vi "MC_Sensor View Window 2.vi"(10 "SRV In":refnum<k5>, 11 "Sensors Config File Path":path) -> (0 "error out":errorcluster)   [LabVIEW 2014]
doc: "Save a renamed copy of this template to a location of your choice. Set \"Sensor Window Filepath\" in your System Config to point to your copy of the Sensor Window.\n\nSet \"Make All Visible\" (located just below the SensorPalette) to TRUE and run this VI directly from its own Run Arrow one time in order to make all the controls visible so that you can move controls around on the front panel. If there are sensors you will not be using, move them out of the frame off to the right (onto the SensorPalette image).\n\nSensorView Window frame should be 746x706. Check this by clicking arrow mouse over bottom right corner of frame. The window will resize to the frame at runtime.\n\nTo place IMAGE ON THE FRONT PANEL, go to Edit >> Import Picture to Clipboard (this works better in LabVIEW rather than copying to clipboard from another application). Then you can paste (Ctrl+V) the image on the front panel. It is recommended to then select your image and select Move To Back (Ctrl+Shift+J) so that sensors are on top if there is any overlap between sensors and your image.\n\n\nAuthor: Mike Schultz (mschultz11711@gmail.com)"
uses:
  SRV VIs/Sensors/SRV_Sensor View refs.ctl
  SRV VIs/Sensors/SRV_Sensor Config Cluster.ctl
  SRV VIs/Sensors/SRV_Sensor Analog-Digital.ctl
  SRV VIs/Sensors/SRV_Sensor Sampling Mode.ctl
  SRV VIs/Sensors/SRV_Sensor View Config Cluster.ctl
  SRV VIs/Sensors/SRV_Sensors Names.ctl
  SRV VIs/Sensors/SRV_Sensor PicoC Shared Var Type.ctl
  SRV VIs/Sensors/SRV_Sensor Number of Bytes.ctl
  SRV VIs/Sensors/SRV_Sensor Integer Word Type.ctl
  SRV VIs/Sensors/SRV_Sensor Config-Command Cluster.ctl
  SRV VIs/Sensors/SRV_Calculated Sensor Cfg.ctl
  SRV VIs/Support/SRV_Command-Data Queue Data Type.ctl
  SRV VIs/Sensors/SRV_Sensor-Value Cluster.ctl
  <vilib>/Utility/error.llb/DialogType.ctl
panel:
  in  "Make All Visible":bool
  out "Overflow Indicator":bool
  out "# elements in queue":i32
  out "Command":string
  in  "Poll":bool
  out "Boolean 32":bool
  out "Boolean 31":bool
  out "Boolean 30":bool
  out "Boolean 29":bool
  out "Boolean 28":bool
  out "Boolean 27":bool
  out "Boolean 26":bool
  out "Boolean 25":bool
  out "Boolean 24":bool
  out "Boolean 23":bool
  out "Boolean 22":bool
  out "Boolean 21":bool
  out "Boolean 20":bool
  out "Boolean 19":bool
  out "Boolean 18":bool
  out "Boolean 17":bool
  out "Boolean 16":bool
  out "Boolean 15":bool
  out "Boolean 14":bool
  out "Boolean 13":bool
  out "Boolean 12":bool
  out "Boolean 11":bool
  out "Boolean 10":bool
  out "Boolean 09":bool
  out "Boolean 08":bool
  out "Boolean 07":bool
  out "Boolean 06":bool
  out "Boolean 05":bool
  out "Boolean 04":bool
  out "Boolean 03":bool
  out "Boolean 02":bool
  out "Boolean 01":bool
  out "Numeric 08":dbl
  out "Numeric 07":dbl
  out "Numeric 06":dbl
  out "Numeric 05":dbl
  out "Numeric 04":dbl
  out "Numeric 03":dbl
  out "Numeric 02":dbl
  out "Numeric 01":dbl
  out "Meter 04":dbl(knob)
  out "Meter 03":dbl(knob)
  out "Meter 02":dbl(knob)
  out "Meter 01":dbl(knob)
  out "Gauge 04":dbl(knob)
  out "Gauge 03":dbl(knob)
  out "Gauge 02":dbl(knob)
  out "Gauge 01":dbl(knob) scale format="%#.3g"
  # "SensorView Window"
  # "SensorPalette"
  # "SensorView Window Instructions\n\nUse the Arrow tool from the Tools Pallet to select, pull and place sensors into the SensorView Window. If you want to remove a sensor from the SensorView Window use the Arrow tool to select and pull the sensor back to the SensorPallet.\n\nTo open the Tools Pallet go to View/Tools Pallet in the standard tool bar. Be sure to close the Tools Pallet when you are finished creating your sensor dashboard.\n\n\n* BE SURE TO PLACE SENSORS BACK IN THEIR CORRECT LOCATION ON THE SENSORPALLET OR YOU WILL END UP WITH A MESS."
  # "Set to TRUE and run this VI directly from its own Run Arrow \none time in order to make all the controls visible so that \nyou can move controls around on the front panel.  If there \nare sensors you will not be using, move them out of the \nframe off to the right."
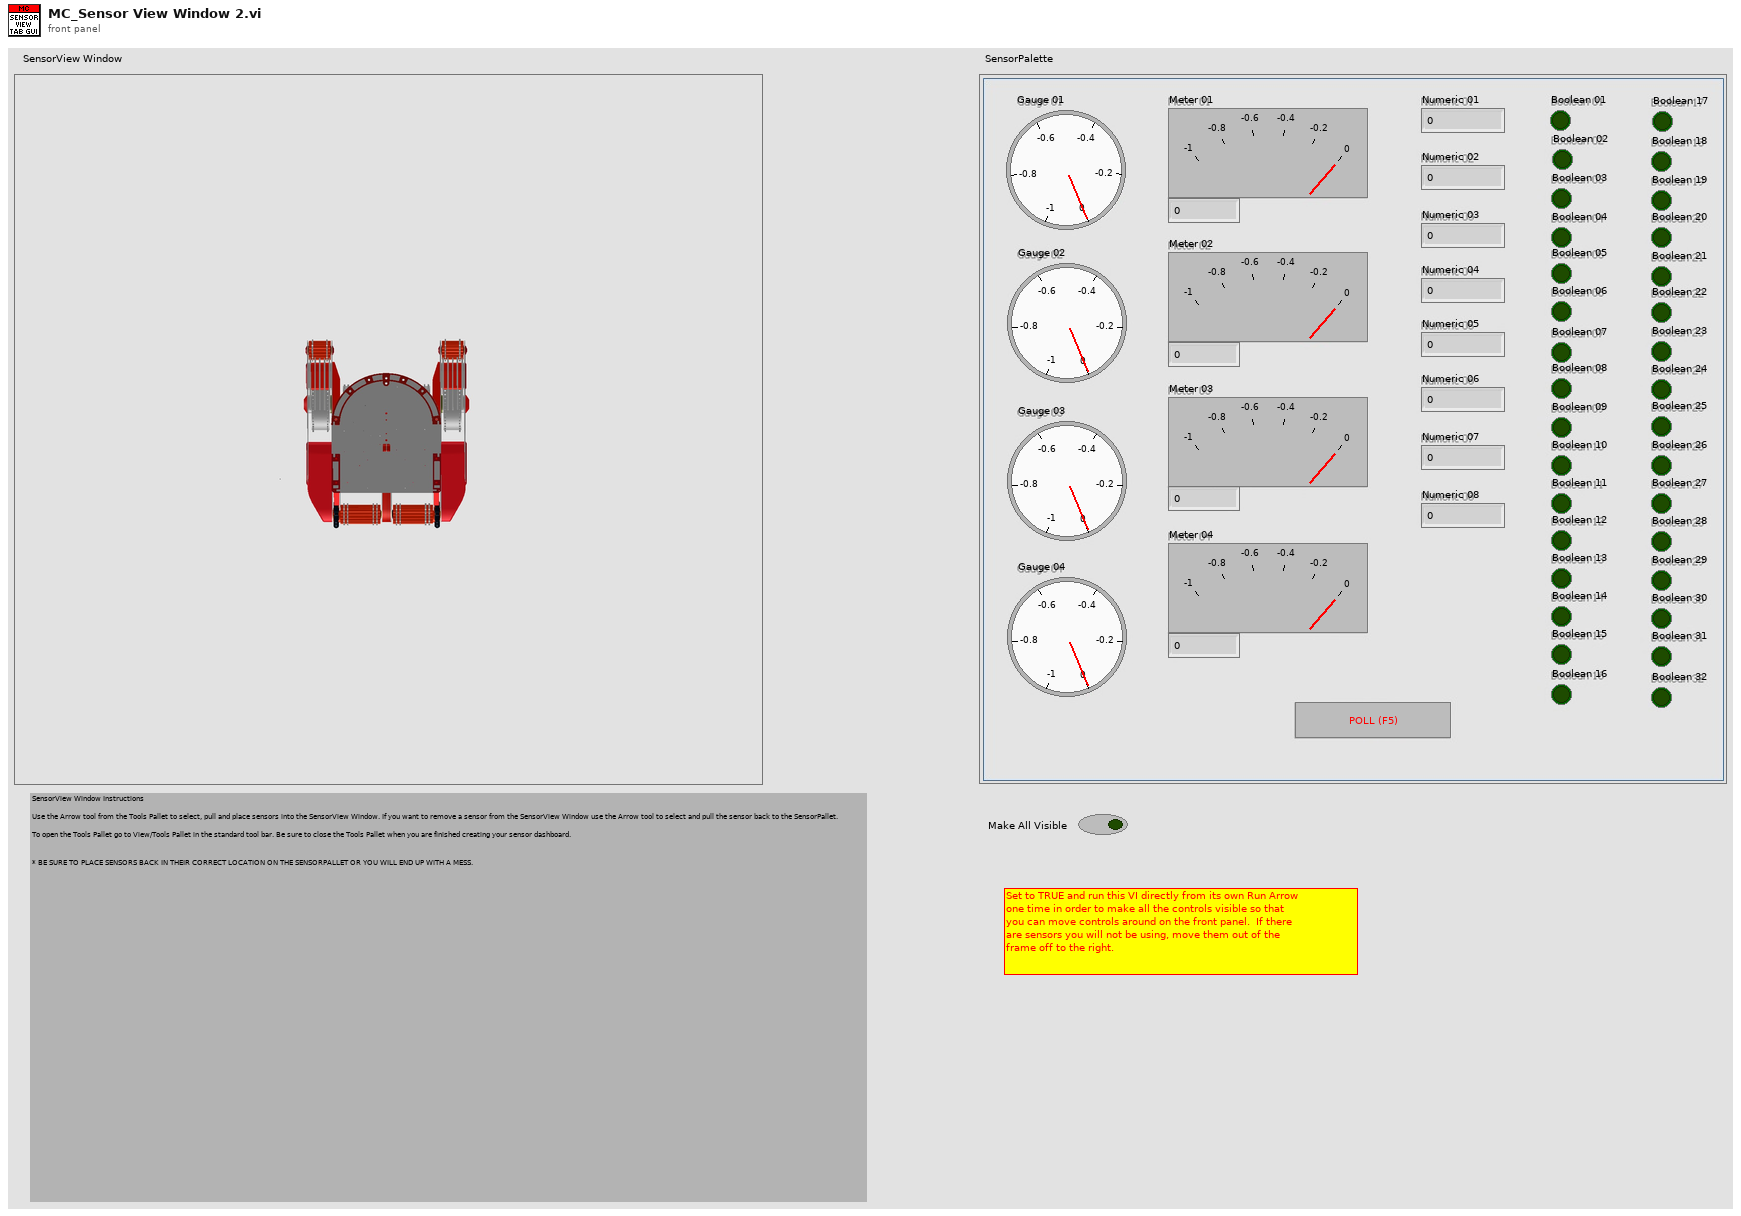
[diagram p1: front panel]
types:
  T1 = typedef "SRV_Command-Data Queue Data Type.ctl" = cluster{"Command":string, "Data":variant}
  T2 = typedef "SRV_Sensor View refs.ctl" = cluster{"Knob refs":refnum<vi>[], "Numeric refs":refnum<vi>[], "Boolean refs":refnum<vi>[]}
  T3 = typedef "SRV_Sensor Config Cluster.ctl" = cluster{"Name":string, "A/D":T4, "I2C Address":u8, "Register":u8, "Channel":u8, "Digital Mask":u16, "Units":string, "Sampling Mode":T5, "Sample Period (ms)":u32, "Formula":string, "Sensor View Config":T6, "Active":bool, "PicoC Shared Var Type":T8, "Index":u8, "Stream Multiple?":bool, "Index End":u8, "Bytes":T9, "Source Sensor Name":string, "Repeat Start":bool, "Integer Word Type":T10, "Byte Swap":bool}
  T4 = typedef "SRV_Sensor Analog-Digital.ctl" = enum16{"Digital", "Analog", "PicoC Shared", "Calculated"}
  T5 = typedef "SRV_Sensor Sampling Mode.ctl" = enum16{"Polled", "Streaming"}
  T6 = typedef "SRV_Sensor View Config Cluster.ctl" = cluster{"Sensor Name":T7, "Minimum":dbl, "Maximum":dbl}
  T7 = typedef "SRV_Sensors Names.ctl" = enum16{"Gauge 01", "Gauge 02", "Gauge 03", "Gauge 04", "Meter 01", "Meter 02", "Meter 03", "Meter 04", "Numeric 01", "Numeric 02", "Numeric 03", "Numeric 04", "Numeric 05", "Numeric 06", "Numeric 07", "Numeric 08", "Boolean 01", "Boolean 02", "Boolean 03", "Boolean 04", "Boolean 05", "Boolean 06", "Boolean 07", "Boolean 08", "Boolean 09", "Boolean 10", "Boolean 11", "Boolean 12", "Boolean 13", "Boolean 14", "Boolean 15", "Boolean 16", "Boolean 17", "Boolean 18", "Boolean 19", "Boolean 20", "Boolean 21", "Boolean 22", "Boolean 23", "Boolean 24", "Boolean 25", "Boolean 26", "Boolean 27", "Boolean 28", "Boolean 29", "Boolean 30", "Boolean 31", "Boolean 32"}
  T8 = typedef "SRV_Sensor PicoC Shared Var Type.ctl" = enum16{"String", "Integer", "Float"}
  T9 = typedef "SRV_Sensor Number of Bytes.ctl" = enum16{"1 Byte", "2 Bytes"}
  T10 = typedef "SRV_Sensor Integer Word Type.ctl" = enum32{"Unsigned", "Signed"}
  T11 = typedef "SRV_Sensor Config-Command Cluster.ctl" = cluster{"Sensor Config":T3, "Command":string, "Parsed Formula":cluster{"Table":i32[][], "Y Values":dbl[]}, "Calculated Sensors Array":T12[]}
  T12 = typedef "SRV_Calculated Sensor Cfg.ctl" = cluster{"Sensor Config":T3, "Parsed Formula":cluster{"Table":i32[][], "Y Values":dbl[]}}
  T13 = cluster{"user event":refnum<user-event>, "Version":string, "Sensor View refs":T2, "This VI ref":refnum<vi>, "Sensors Config File Path":path, "Sensors Config":T3[], "SRV ref":refnum<k5>, "Streaming Cfg-Cmds":T11[], "Polled Cfg-Cmds":T11[], "Off Cfg-Cmds":T11[], "Streaming Sensor View Indicator Names":T7[], "Polled Sensor View Indicator Names":T7[], "Make All Visible":bool}
  T14 = typedef "SRV_Sensor-Value Cluster.ctl" = cluster{"Sensor Name":T7, "Value":dbl}
  T15 = typedef "DialogType.ctl" = u16
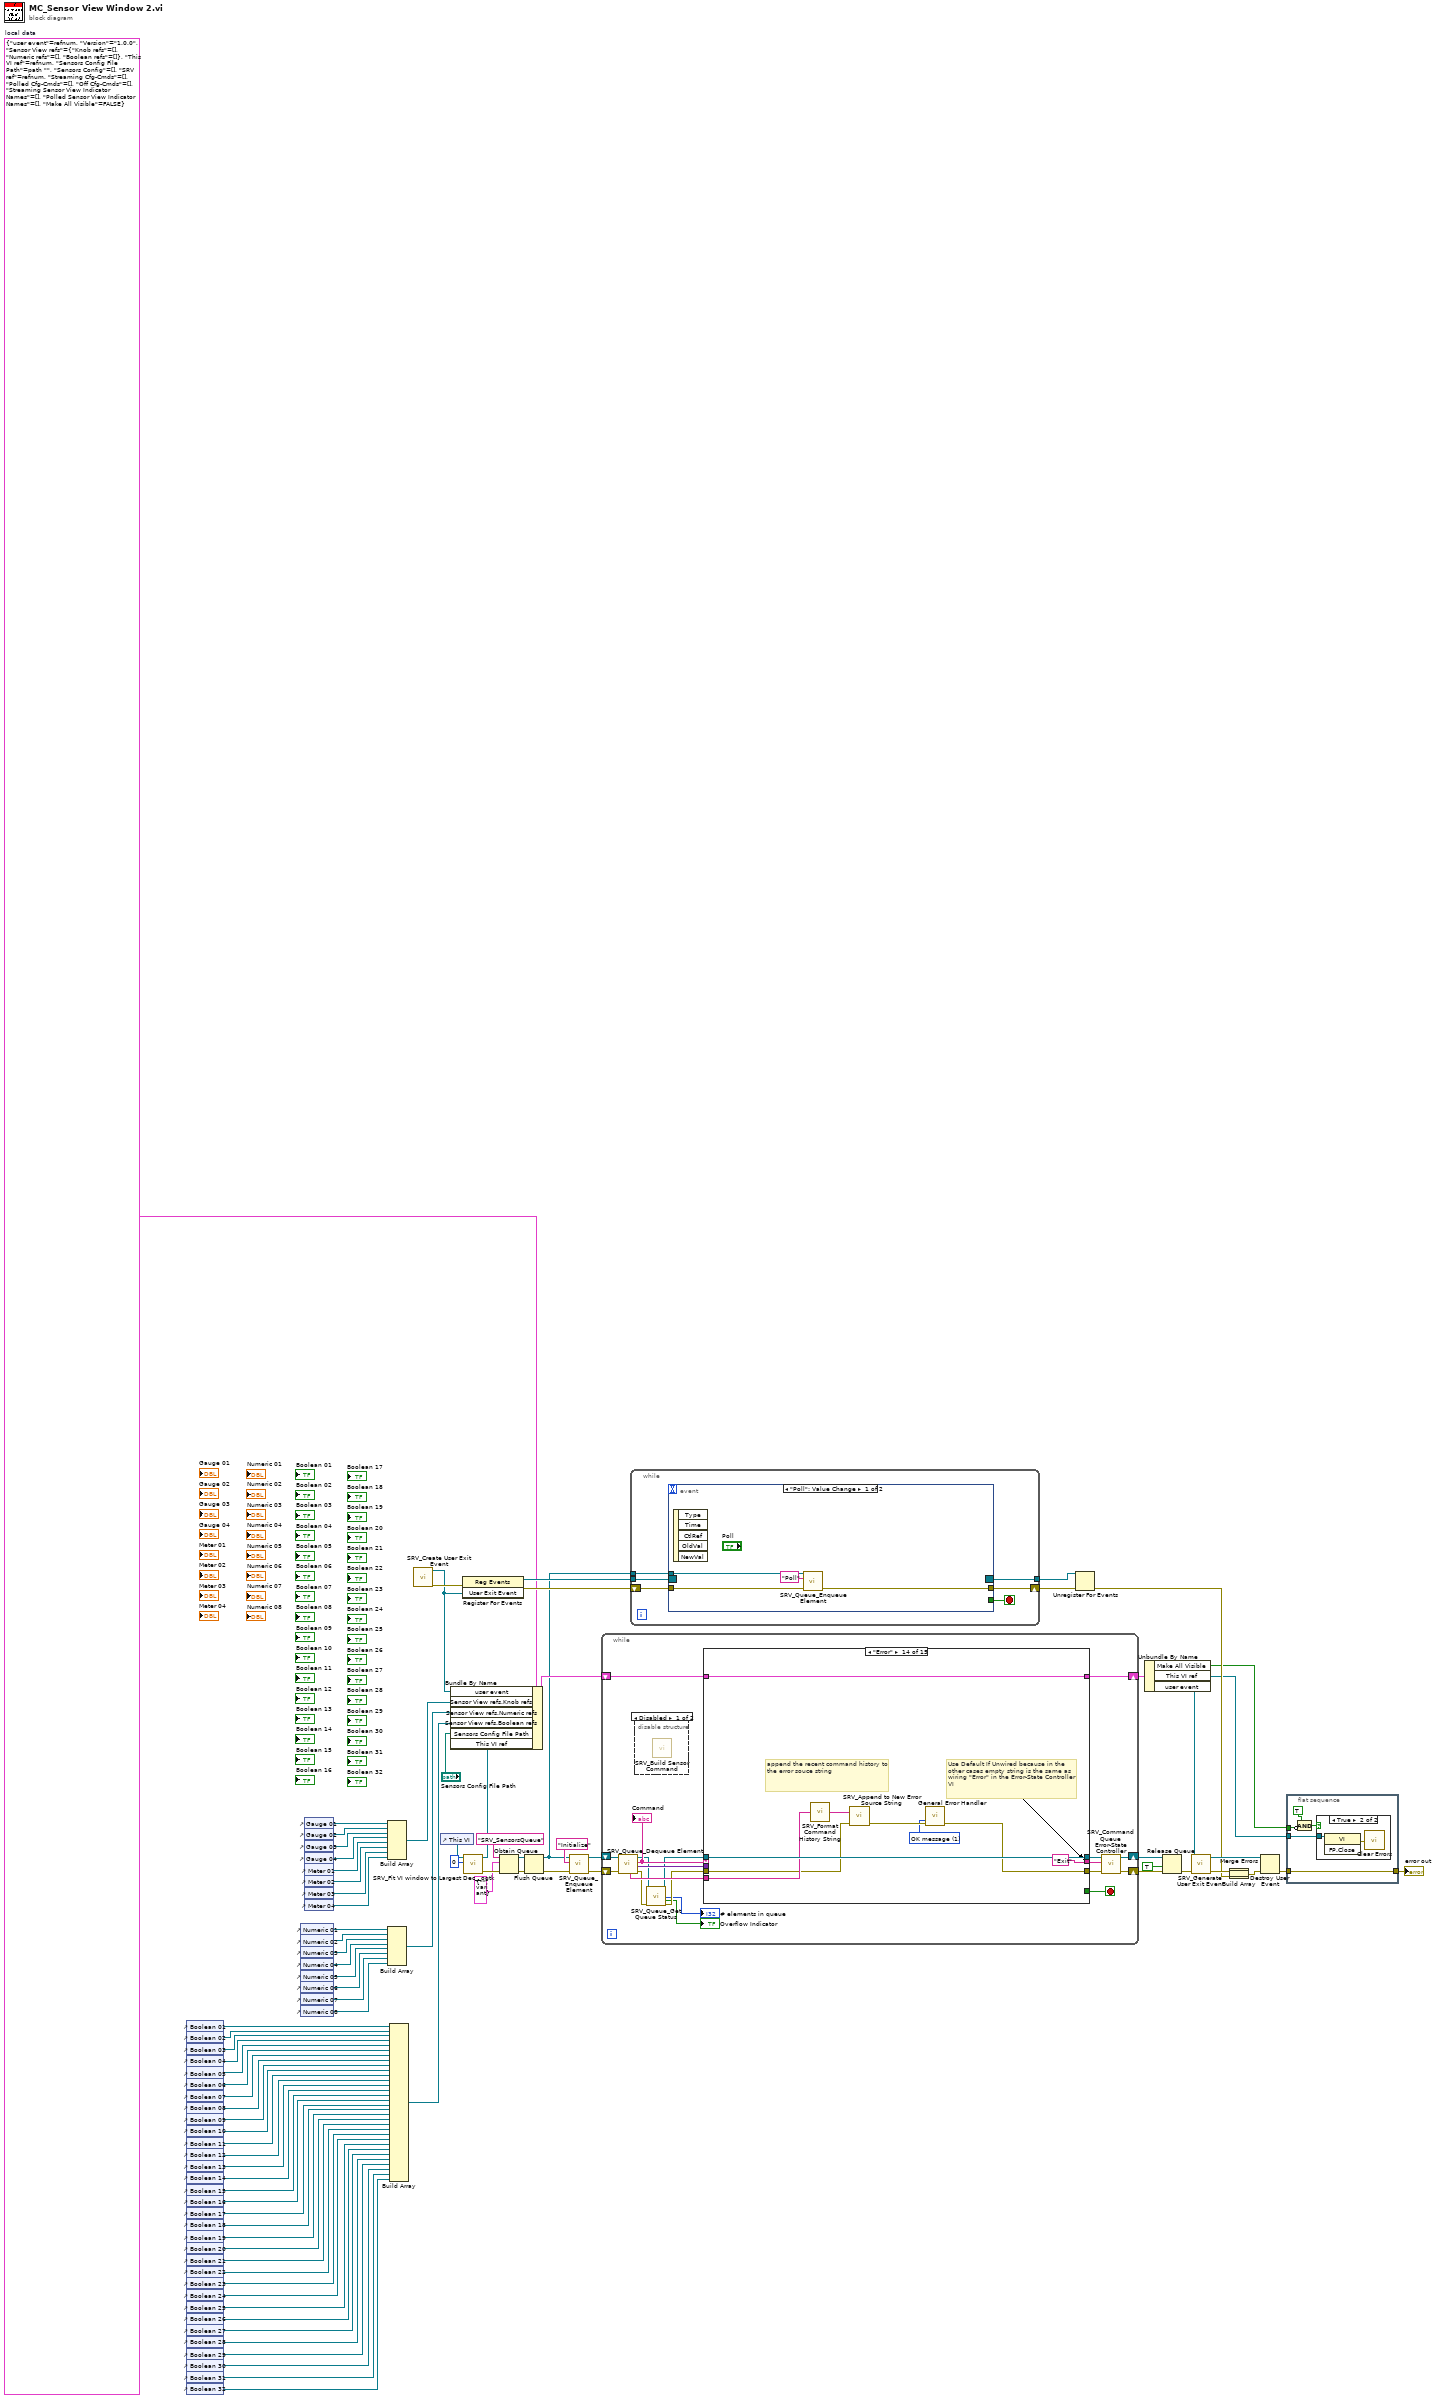
[diagram p0: block diagram]
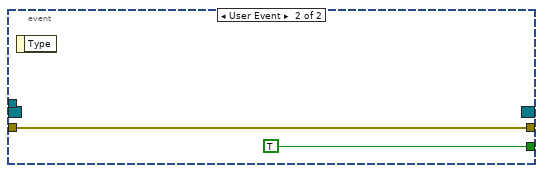
[diagram p3: hidden frame]
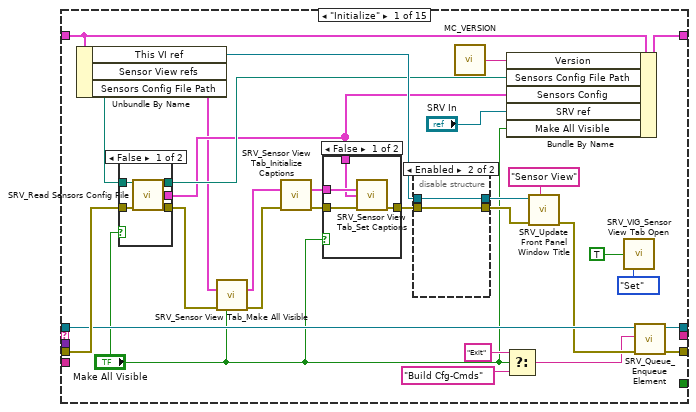
[diagram p5: hidden frame]
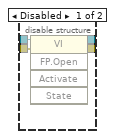
[diagram p6: hidden frame]
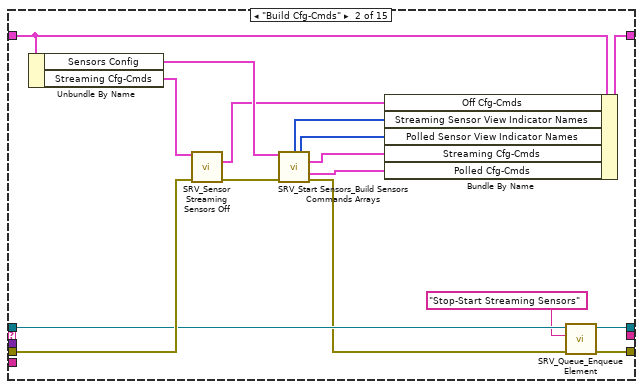
[diagram p9: hidden frame]
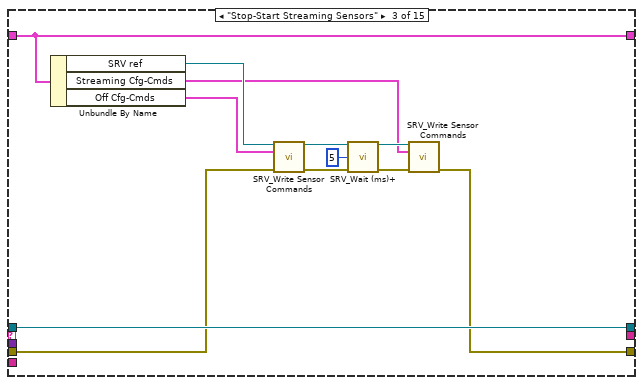
[diagram p10: hidden frame]
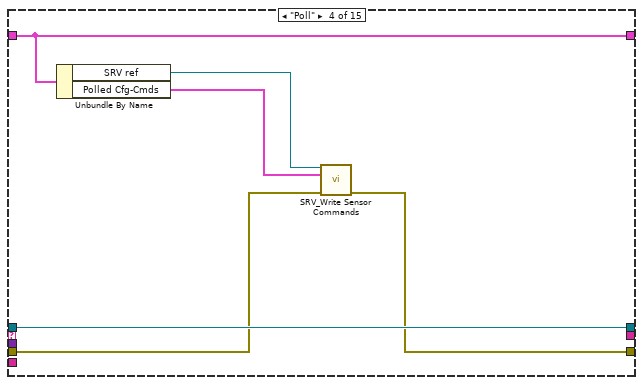
[diagram p11: hidden frame]
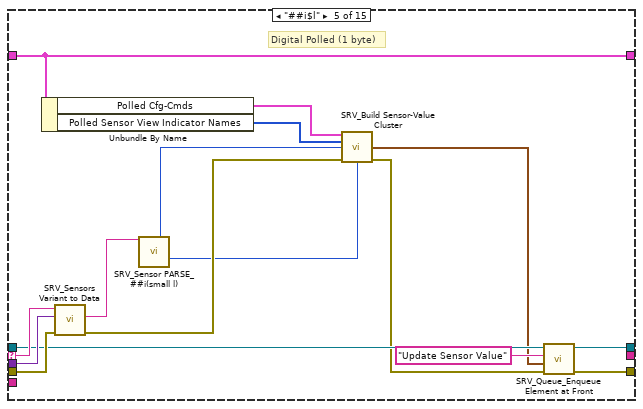
[diagram p12: hidden frame]
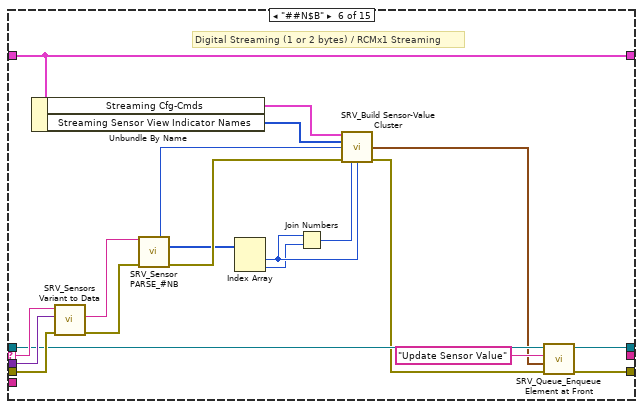
[diagram p13: hidden frame]
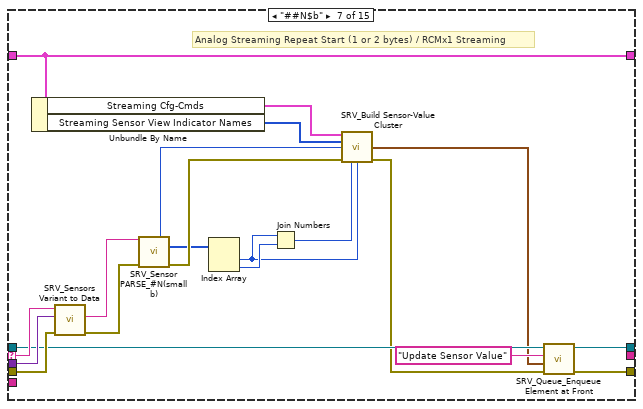
[diagram p14: hidden frame]
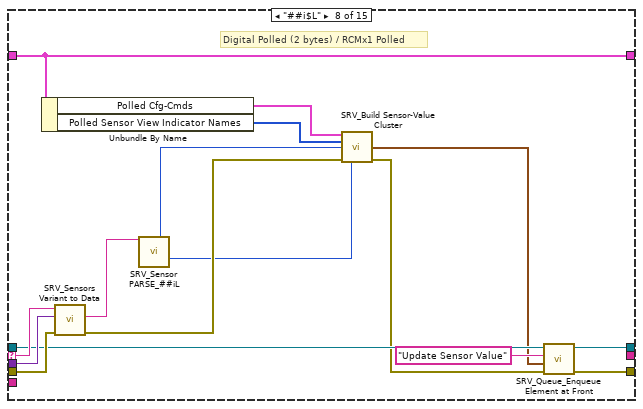
[diagram p15: hidden frame]
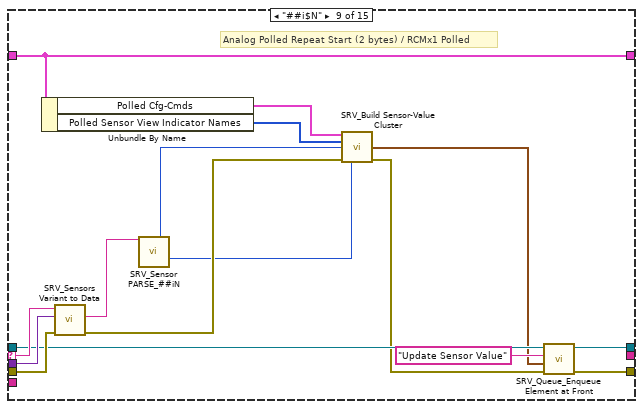
[diagram p16: hidden frame]
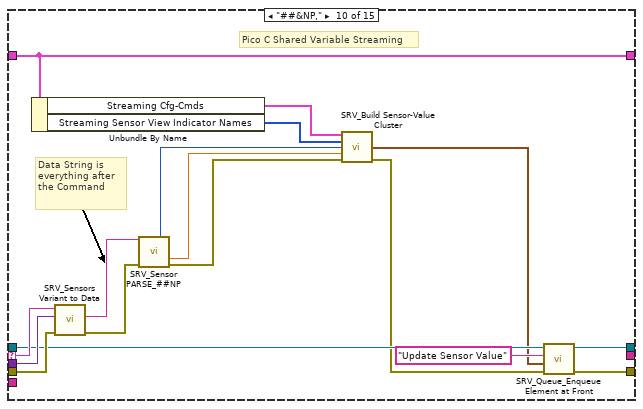
[diagram p17: hidden frame]
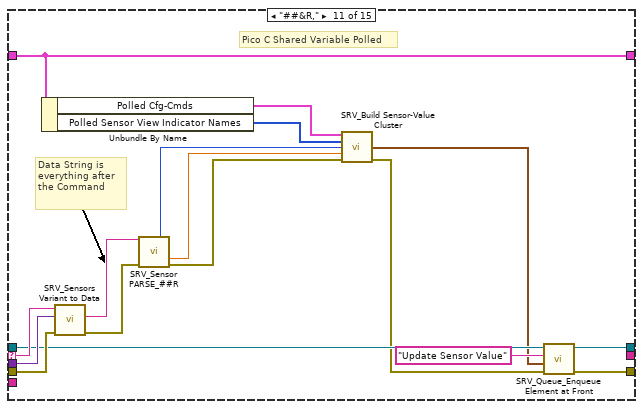
[diagram p18: hidden frame]
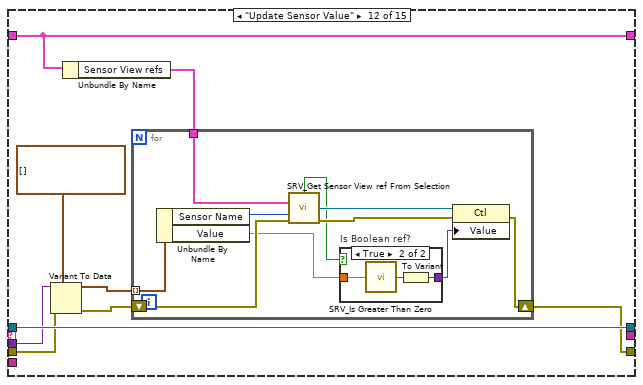
[diagram p19: hidden frame]
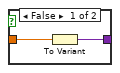
[diagram p20: hidden frame]
diagram:
  w82 = T13 {"user event"=refnum, "Version"="1.0.0", "Sensor View refs"={"Knob refs"=[], "Numeric refs"=[], "Boolean refs"=[]}, "This VI ref"=refnum, "Sensors Config File Path"=path "", "Sensors Config"=[], "SRV ref"=refnum, "Streaming Cfg-Cmds"=[], "Polled Cfg-Cmds"=[], "Off Cfg-Cmds"=[], "Streaming Sensor View Indicator Names"=[], "Polled Sensor View Indicator Names"=[], "Make All Visible"=FALSE}  # local data
  n1 = control-ref of="Boolean 01"() -> (w49:refnum<vi>)
  n2 = control-ref of="Boolean 02"() -> (w48:refnum<vi>)
  n3 = control-ref of="Boolean 03"() -> (w47:refnum<vi>)
  n4 = control-ref of="Boolean 04"() -> (w46:refnum<vi>)
  n5 = control-ref of="Boolean 05"() -> (w45:refnum<vi>)
  n6 = control-ref of="Boolean 06"() -> (w44:refnum<vi>)
  n7 = control-ref of="Boolean 07"() -> (w43:refnum<vi>)
  n8 = control-ref of="Boolean 08"() -> (w42:refnum<vi>)
  n9 = control-ref of="Boolean 09"() -> (w41:refnum<vi>)
  n10 = control-ref of="Boolean 10"() -> (w40:refnum<vi>)
  n11 = control-ref of="Boolean 11"() -> (w39:refnum<vi>)
  n12 = control-ref of="Boolean 12"() -> (w38:refnum<vi>)
  n13 = control-ref of="Boolean 13"() -> (w37:refnum<vi>)
  n14 = control-ref of="Boolean 14"() -> (w36:refnum<vi>)
  n15 = control-ref of="Boolean 15"() -> (w35:refnum<vi>)
  n16 = control-ref of="Boolean 16"() -> (w34:refnum<vi>)
  n17 = control-ref of="Boolean 17"() -> (w33:refnum<vi>)
  n18 = control-ref of="Boolean 18"() -> (w32:refnum<vi>)
  n19 = control-ref of="Boolean 19"() -> (w31:refnum<vi>)
  n20 = control-ref of="Boolean 20"() -> (w30:refnum<vi>)
  n21 = control-ref of="Boolean 21"() -> (w29:refnum<vi>)
  n22 = control-ref of="Boolean 22"() -> (w28:refnum<vi>)
  n23 = control-ref of="Boolean 23"() -> (w27:refnum<vi>)
  n24 = control-ref of="Boolean 24"() -> (w26:refnum<vi>)
  n25 = control-ref of="Boolean 25"() -> (w25:refnum<vi>)
  n26 = control-ref of="Boolean 26"() -> (w24:refnum<vi>)
  n27 = control-ref of="Boolean 27"() -> (w23:refnum<vi>)
  n28 = control-ref of="Boolean 28"() -> (w22:refnum<vi>)
  n29 = control-ref of="Boolean 29"() -> (w21:refnum<vi>)
  n30 = control-ref of="Boolean 30"() -> (w20:refnum<vi>)
  n31 = control-ref of="Boolean 31"() -> (w19:refnum<vi>)
  n32 = control-ref of="Boolean 32"() -> (w18:refnum<vi>)
  n33 = control-ref of="Numeric 01"() -> (w57:refnum<vi>)
  n34 = control-ref of="Numeric 02"() -> (w56:refnum<vi>)
  n35 = control-ref of="Numeric 03"() -> (w55:refnum<vi>)
  n36 = control-ref of="Numeric 04"() -> (w54:refnum<vi>)
  n37 = control-ref of="Numeric 05"() -> (w53:refnum<vi>)
  n38 = control-ref of="Numeric 06"() -> (w52:refnum<vi>)
  n39 = control-ref of="Numeric 07"() -> (w51:refnum<vi>)
  n40 = control-ref of="Numeric 08"() -> (w50:refnum<vi>)
  n41 = control-ref of="Gauge 01"() -> (w65:refnum<vi>)
  n42 = control-ref of="Gauge 02"() -> (w64:refnum<vi>)
  n43 = control-ref of="Gauge 03"() -> (w63:refnum<vi>)
  n44 = control-ref of="Gauge 04"() -> (w62:refnum<vi>)
  n45 = control-ref of="Meter 01"() -> (w61:refnum<vi>)
  n46 = control-ref of="Meter 02"() -> (w60:refnum<vi>)
  n47 = control-ref of="Meter 03"() -> (w59:refnum<vi>)
  n48 = control-ref of="Meter 04"() -> (w58:refnum<vi>)
  n49 = Build Array(w65, w64, w63, w62, w61, w60, w59, w58) -> (w12:refnum<vi>[])
  n50 = Build Array(w57, w56, w55, w54, w53, w52, w51, w50) -> (w13:refnum<vi>[])
  n51 = Build Array(w49, w48, w47, w46, w45, w44, w43, w42, w41, w40, w39, w38, w37, w36, w35, w34, w33, w32, w31, w30, w29, w28, w27, w26, w25, w24, w23, w22, w21, w20, w19, w18) -> (w14:refnum<vi>[])
  n52 = call "SRV_Create User Exit Event.vi"() -> ("error out"=w73:errorcluster, "User Exit Event"=w72:refnum<user-event>)  [unwired: 10 in]
  n53 = control-ref of="This VI"() -> (w3:refnum<vi>)
  n54 = register-events(error in=w73, w72) -> (reference out=w88:refnum<event-registration>, error out=w87:errorcluster)  [unwired: 1 in]
  n55 = call "SRV_Fit VI window to Largest Dec__ogtk.vi"("border spacing (2 px)"=0, "VI Ref (calling VI)"=w3) -> ("error out"=w68:errorcluster, "dup VI Ref"=w11:refnum<vi>)  [unwired: 4 in]
  n56 = Bundle By Name(cluster=w82, "user event"=w72, "Sensor View refs.Knob refs"=w12, "Sensor View refs.Numeric refs"=w13, "Sensor View refs.Boolean refs"=w14, "Sensors Config File Path"="Sensors Config File Path", "This VI ref"=w11) -> (w81:T13)
  n57 = Obtain Queue(name (unnamed)="SRV_SensorsQueue", element data type=T1 {"Command"="", "Data"=variant} ("Queue Data Type"), error in (no error)=w68) -> (queue out=w5:refnum<queue>, error out=w7:errorcluster)  [unwired: 2 in, 1 out]
  n58 = Flush Queue(queue=w5, error in (no error)=w7) -> (queue out=w4:refnum<queue>, error out=w6:errorcluster)  [unwired: 1 out]
  n59 = call "SRV_Queue_Enqueue Element.vi"("error in (no error)"=w6, "Command"="Initialize", "Command-Data Queue"=w4) -> ("error out"=w66:errorcluster, "Command-Data Queue out"=w69:refnum<queue>)  [unwired: 6 in, 1 out]
  n60 = while {
    shift-right: [w103] -> w84
    shift-left: w66 -> [w107]
    shift-right: [w101] -> w83
    shift-left: w69 -> [w106]
    shift-right: [w95] -> w80
    shift-left: w81 -> [w96]
    stop <- w97 stop-if-true
    n61 = call "SRV_Queue_Dequeue Element.vi"("error in (no error)"=w107, "Command-Data Queue"=w106) -> ("error out"=w94:errorcluster, "Data"=w100:variant, "Command"=w105:string, "Command-Data Queue out"=w92:refnum<queue>, "Command History"=w99:string[])  [unwired: 4 in, 1 out]
    "Command" <- w105
    n62 = disable-structure shown="Disabled" {
      frame Disabled {
        n63 = call "SRV_Build Sensor Command.vi"() -> ()  [unwired: 10 in, 6 out]
      }
      frame Enabled {
      }
    }
    n64 = call "SRV_Queue_Get Queue Status.vi"("Command-Data Queue"=w92, "error in (no error)"=w94) -> ("Command-Data Queue out"=w91:refnum<queue>, "# elements in queue"=→"# elements in queue":i32, "Overflow Indicator"=→"Overflow Indicator":bool, "error out"=w93:errorcluster)  [unwired: 10 in]
    n65 = case shown="\"Error\"" w105 {
      selector: w105 -> [_ _ _ _ w202 w222 w242 w258 w274 w291 w308 _ w338 _ _]
      tunnel: w93 -> [w135 w164 w179 w183 w201 w221 w241 w257 w273 w290 w307 w317 w336 w345 w352]
      tunnel: [w125 w159 w174 w182 w191 w212 w232 w247 w263 w280 w297 w311 w335 w342 w351] -> w104
      tunnel: w91 -> [w127 w161 w180 w187 w194 w215 w235 w250 w266 w283 w300 w318 w340 w349 w362]
      tunnel: [w126 w160 w180 w187 w193 w214 w234 w249 w265 w282 w299 w318 w340 w349 w362] -> w102
      tunnel: w100 -> [_ _ _ _ w203 w223 w243 w259 w275 w292 w309 w316 _ _ _]
      tunnel: w99 -> [_ _ _ _ _ _ _ _ _ _ _ _ _ w348 _]
      tunnel: [_ _ _ _ _ _ _ _ _ _ _ _ _ "Exit" ("Error Command") _] -> w98
      tunnel: [_ _ _ _ _ _ _ _ _ _ _ _ _ _ TRUE] -> w97
      tunnel: w96 -> [w114 w169 w181 w186 w199 w219 w239 w255 w271 w288 w305 w315 w337 w346 w358]
      tunnel: [w136 w168 w181 w186 w199 w219 w239 w255 w271 w288 w305 w315 w337 w346 w358] -> w95
      frame "Initialize" {
        n66 = Unbundle By Name(w114) -> ("This VI ref"=w132:refnum<vi>, "Sensor View refs"=w113:T2, "Sensors Config File Path"=w129:path)
        n67 = case shown="False" "Make All Visible" {
          tunnel: w135 -> [w147 w148]
          tunnel: [w146 w149] -> w130
          tunnel: w129 -> [w145 w149]
          tunnel: [w144 _] -> w128
          tunnel: [w143 w148] -> w116
          frame False {
            n68 = call "SRV_Read Sensors Config File.vi"("Sensors Config File Path"=w145, "error in (no error)"=w147) -> ("Sensors Config File Path out"=w146:path, "Sensors Config"=w144:T3[], "error out"=w143:errorcluster)  [unwired: 10 in, 1 out]
          }
          frame True {
          }
        }
        n69 = call "SRV_Sensor View Tab_Make All Visible.vi"("Sensor View refs"=w113, "error in (no error)"=w116, "Make All Visible?"="Make All Visible") -> ("Sensor View refs dup"=w112:T2, "error out"=w115:errorcluster)  [unwired: 11 in]
        n70 = call "SRV_Sensor View Tab_Initialize Captions.vi"("Sensor View refs"=w112, "error in (no error)"=w115) -> ("Sensor View refs dup"=w133:T2, "error out"=w134:errorcluster)  [unwired: 12 in]
        n71 = case shown="False" "Make All Visible" {
          tunnel: w134 -> [w153 w154]
          tunnel: w133 -> [w152 _]
          tunnel: [w151 w154] -> w131
          tunnel: w128 -> [w150 _]
          frame False {
            n72 = call "SRV_Sensor View Tab_Set Captions.vi"("Sensor View refs"=w152, "Sensors Config"=w150, "error in (no error)"=w153) -> ("error out"=w151:errorcluster)  [unwired: 11 in, 1 out]
          }
          frame True {
          }
        }
        n73 = disable-structure shown="Enabled" {
          disable-tunnel: w132 -> [w140 w142]
          disable-tunnel: w131 -> [w139 w141]
          disable-tunnel: [w138 w141] -> w122
          disable-tunnel: [w137 w142] -> w121
          frame Disabled {
            n74 = invoke class="VI" method="FP.Open"(reference=w140, error in=w139) -> (reference out=w137:refnum<vi>, error out=w138:errorcluster)  [unwired: 3 in, 3 out]
          }
          frame Enabled {
          }
        }
        n75 = call "MC_VERSION.vi"() -> ("MC Version"=w123:string)
        n76 = Bundle By Name(cluster=w114, "Version"=w123, "Sensors Config File Path"=w130, "Sensors Config"=w128, "SRV ref"="SRV In", "Make All Visible"="Make All Visible") -> (w136:T13)
        n77 = Select(t="Exit", s="Make All Visible", f="Build Cfg-Cmds" ("Command")) -> (s? t:f=w111:string)
        n78 = call "SRV_Update Front Panel Window Title.vi"("Window Title Override String"="Sensor View", "error in (no error)"=w122, "VI ref"=w121) -> ("error out"=w120:errorcluster)  [unwired: 7 in, 1 out]
        n79 = call "SRV_VIG_Sensor View Tab Open.vi"("Sensor View Tab Open"=TRUE, "Method (Get)"=enum16{"Get", "Set"}."Set") -> ()  [unwired: 12 in, 2 out]
        n80 = call "SRV_Queue_Enqueue Element.vi"("error in (no error)"=w120, "Command"=w111, "Command-Data Queue"=w127) -> ("error out"=w125:errorcluster, "Command-Data Queue out"=w126:refnum<queue>)  [unwired: 6 in, 1 out]
      }
      frame "Build Cfg-Cmds" {
        n81 = Unbundle By Name(w169) -> ("Sensors Config"=w170:T3[], "Streaming Cfg-Cmds"=w165:T11[])
        n82 = call "SRV_Sensor Streaming Sensors Off.vi"("Previous Streaming Cfg-Cmds"=w165, "error in (no error)"=w164) -> ("Streaming Cfg-Cmds OFF"=w162:T11[], "error out"=w163:errorcluster)  [unwired: 12 in]
        n83 = call "SRV_Start Sensors_Build Sensors Commands Arrays.vi"("Sensors Config"=w170, "error in (no error)"=w163) -> ("Streaming Sensor View Indicator Names"=w156:T7[], "Polled Sensor View Indicator Names"=w155:T7[], "Active Streaming Cfg-Commands"=w167:T11[], "Active Polled Cfg-Commands"=w166:T11[], "error out"=w158:errorcluster)  [unwired: 9 in]
        n84 = Bundle By Name(cluster=w169, "Off Cfg-Cmds"=w162, "Streaming Sensor View Indicator Names"=w156, "Polled Sensor View Indicator Names"=w155, "Streaming Cfg-Cmds"=w167, "Polled Cfg-Cmds"=w166) -> (w168:T13)
        n85 = call "SRV_Queue_Enqueue Element.vi"("error in (no error)"=w158, "Command"="Stop-Start Streaming Sensors", "Command-Data Queue"=w161) -> ("error out"=w159:errorcluster, "Command-Data Queue out"=w160:refnum<queue>)  [unwired: 6 in, 1 out]
      }
      frame "Stop-Start Streaming Sensors" {
        n86 = Unbundle By Name(w181) -> ("SRV ref"=w178:refnum<k5>, "Streaming Cfg-Cmds"=w175:T11[], "Off Cfg-Cmds"=w177:T11[])
        n87 = call "SRV_Write Sensor Commands.vi"("SRV In"=w178, "Sensor Cfg-Commands"=w177, "error in (no error)"=w179) -> ("SRV out"=w176:refnum<k5>, "error out"=w173:errorcluster)  [unwired: 11 in]
        n88 = call "SRV_Wait (ms)+.vi"("milliseconds to wait"=u32 5, "error in (no error)"=w173) -> ("error out"=w172:errorcluster)  [unwired: 12 in, 1 out]
        n89 = call "SRV_Write Sensor Commands.vi"("SRV In"=w176, "Sensor Cfg-Commands"=w175, "error in (no error)"=w172) -> ("error out"=w174:errorcluster)  [unwired: 11 in, 1 out]
      }
      frame "Poll" {
        n90 = Unbundle By Name(w186) -> ("SRV ref"=w184:refnum<k5>, "Polled Cfg-Cmds"=w185:T11[])
        n91 = call "SRV_Write Sensor Commands.vi"("SRV In"=w184, "Sensor Cfg-Commands"=w185, "error in (no error)"=w183) -> ("error out"=w182:errorcluster)  [unwired: 11 in, 1 out]
      }
      frame "##i$l" {
        # "Digital Polled (1 byte)"
        n92 = Unbundle By Name(w199) -> ("Polled Cfg-Cmds"=w198:T11[], "Polled Sensor View Indicator Names"=w197:T7[])
        n93 = call "SRV_Sensors Variant to Data.vi"("error in (no error)"=w201, "Data"=w203, "Command"=w202) -> ("error out"=w195:errorcluster, "Data String"=w200:string)  [unwired: 7 in]
        n94 = call "SRV_Sensor PARSE_##i(small l).vi"("Return Data"=w200) -> ("Sensor View Indicator Names"=w196:T7, "Value"=w188:u8)  [unwired: 13 in]
        n95 = call "SRV_Build Sensor-Value Cluster.vi"("Cfg-Cmds"=w198, "Sensor View Indicator Names"=w197, "Sensor View Indicator Name"=w196, "error in (no error)"=w195, "Value (U8)"=w188) -> ("Array of Sensor-Value Cluster"=w189:T14[], "error out"=w192:errorcluster)  [unwired: 9 in]
        n96 = call "SRV_Queue_Enqueue Element at Front.vi"("error in (no error)"=w192, "Data"=w189, "Command"="Update Sensor Value", "Command-Data Queue"=w194) -> ("error out"=w191:errorcluster, "Command-Data Queue out"=w193:refnum<queue>)  [unwired: 5 in, 1 out]
      }
      frame "##N$B" {
        # "Digital Streaming (1 or 2 bytes) / RCMx1 Streaming"
        n97 = Unbundle By Name(w219) -> ("Streaming Cfg-Cmds"=w218:T11[], "Streaming Sensor View Indicator Names"=w217:T7[])
        n98 = call "SRV_Sensors Variant to Data.vi"("error in (no error)"=w221, "Data"=w223, "Command"=w222) -> ("error out"=w209:errorcluster, "Data String"=w220:string)  [unwired: 7 in]
        n99 = call "SRV_Sensor PARSE_#NB.vi"("Return Data"=w220, "error in (no error)"=w209) -> ("Sensor View Indicator Names"=w216:T7, "Values (U8)"=w207:u8[], "error out"=w208:errorcluster)  [unwired: 11 in]
        n100 = Index Array(array=w207) -> (element #1=w206:u8, element #2=w205:u8)  [unwired: 2 in]
        n101 = Join Numbers(hi=w206, lo=w205) -> ((hi.lo)=w204:u16)
        n102 = call "SRV_Build Sensor-Value Cluster.vi"("Cfg-Cmds"=w218, "Sensor View Indicator Names"=w217, "Sensor View Indicator Name"=w216, "error in (no error)"=w208, "Value (U16)"=w204, "Value (U8)"=w206) -> ("Array of Sensor-Value Cluster"=w210:T14[], "error out"=w213:errorcluster)  [unwired: 8 in]
        n103 = call "SRV_Queue_Enqueue Element at Front.vi"("error in (no error)"=w213, "Data"=w210, "Command"="Update Sensor Value", "Command-Data Queue"=w215) -> ("error out"=w212:errorcluster, "Command-Data Queue out"=w214:refnum<queue>)  [unwired: 5 in, 1 out]
      }
      frame "##N$b" {
        # "Analog Streaming Repeat Start (1 or 2 bytes) / RCMx1 Streaming"
        n104 = Unbundle By Name(w239) -> ("Streaming Cfg-Cmds"=w238:T11[], "Streaming Sensor View Indicator Names"=w237:T7[])
        n105 = call "SRV_Sensors Variant to Data.vi"("error in (no error)"=w241, "Data"=w243, "Command"=w242) -> ("error out"=w229:errorcluster, "Data String"=w240:string)  [unwired: 7 in]
        n106 = call "SRV_Sensor PARSE_#N(small b).vi"("Return Data"=w240, "error in (no error)"=w229) -> ("Sensor View Indicator Names"=w236:T7, "Values (U8)"=w226:u8[], "error out"=w228:errorcluster)  [unwired: 11 in]
        n107 = Index Array(array=w226) -> (element #1=w224:u8, element #2=w227:u8)  [unwired: 2 in]
        n108 = Join Numbers(hi=w224, lo=w227) -> ((hi.lo)=w225:u16)
        n109 = call "SRV_Build Sensor-Value Cluster.vi"("Cfg-Cmds"=w238, "Sensor View Indicator Names"=w237, "Sensor View Indicator Name"=w236, "error in (no error)"=w228, "Value (U16)"=w225, "Value (U8)"=w224) -> ("Array of Sensor-Value Cluster"=w230:T14[], "error out"=w233:errorcluster)  [unwired: 8 in]
        n110 = call "SRV_Queue_Enqueue Element at Front.vi"("error in (no error)"=w233, "Data"=w230, "Command"="Update Sensor Value", "Command-Data Queue"=w235) -> ("error out"=w232:errorcluster, "Command-Data Queue out"=w234:refnum<queue>)  [unwired: 5 in, 1 out]
      }
      frame "##i$L" {
        # "Digital Polled (2 bytes) / RCMx1 Polled"
        n111 = Unbundle By Name(w255) -> ("Polled Cfg-Cmds"=w254:T11[], "Polled Sensor View Indicator Names"=w253:T7[])
        n112 = call "SRV_Sensors Variant to Data.vi"("error in (no error)"=w257, "Data"=w259, "Command"=w258) -> ("error out"=w251:errorcluster, "Data String"=w256:string)  [unwired: 7 in]
        n113 = call "SRV_Sensor PARSE_##iL.vi"("Return Data"=w256) -> ("Sensor View Indicator Names"=w252:T7, "Value"=w244:u16)  [unwired: 13 in]
        n114 = call "SRV_Build Sensor-Value Cluster.vi"("Cfg-Cmds"=w254, "Sensor View Indicator Names"=w253, "Sensor View Indicator Name"=w252, "error in (no error)"=w251, "Value (U16)"=w244) -> ("Array of Sensor-Value Cluster"=w245:T14[], "error out"=w248:errorcluster)  [unwired: 9 in]
        n115 = call "SRV_Queue_Enqueue Element at Front.vi"("error in (no error)"=w248, "Data"=w245, "Command"="Update Sensor Value", "Command-Data Queue"=w250) -> ("error out"=w247:errorcluster, "Command-Data Queue out"=w249:refnum<queue>)  [unwired: 5 in, 1 out]
      }
      frame "##i$N" {
        # "Analog Polled Repeat Start (2 bytes) / RCMx1 Polled"
        n116 = Unbundle By Name(w271) -> ("Polled Cfg-Cmds"=w270:T11[], "Polled Sensor View Indicator Names"=w269:T7[])
        n117 = call "SRV_Sensors Variant to Data.vi"("error in (no error)"=w273, "Data"=w275, "Command"=w274) -> ("error out"=w267:errorcluster, "Data String"=w272:string)  [unwired: 7 in]
        n118 = call "SRV_Sensor PARSE_##iN.vi"("Return Data"=w272) -> ("Sensor View Indicator Names"=w268:T7, "Value"=w260:u16)  [unwired: 13 in]
        n119 = call "SRV_Build Sensor-Value Cluster.vi"("Cfg-Cmds"=w270, "Sensor View Indicator Names"=w269, "Sensor View Indicator Name"=w268, "error in (no error)"=w267, "Value (U16)"=w260) -> ("Array of Sensor-Value Cluster"=w261:T14[], "error out"=w264:errorcluster)  [unwired: 9 in]
        n120 = call "SRV_Queue_Enqueue Element at Front.vi"("error in (no error)"=w264, "Data"=w261, "Command"="Update Sensor Value", "Command-Data Queue"=w266) -> ("error out"=w263:errorcluster, "Command-Data Queue out"=w265:refnum<queue>)  [unwired: 5 in, 1 out]
      }
      frame "##&NP," {
        # "Data String is everything after the Command"
        # "Pico C Shared Variable Streaming"
        n121 = Unbundle By Name(w288) -> ("Streaming Cfg-Cmds"=w287:T11[], "Streaming Sensor View Indicator Names"=w286:T7[])
        n122 = call "SRV_Sensors Variant to Data.vi"("error in (no error)"=w290, "Data"=w292, "Command"=w291) -> ("error out"=w277:errorcluster, "Data String"=w289:string)  [unwired: 7 in]
        n123 = call "SRV_Sensor PARSE_##NP.vi"("Return Data"=w289, "error in (no error)"=w277) -> ("Sensor View Indicator Names"=w285:T7, "Value"=w284:dbl, "error out"=w276:errorcluster)  [unwired: 11 in]
        n124 = call "SRV_Build Sensor-Value Cluster.vi"("Cfg-Cmds"=w287, "Sensor View Indicator Names"=w286, "Sensor View Indicator Name"=w285, "Value (for Pico C)"=w284, "error in (no error)"=w276) -> ("Array of Sensor-Value Cluster"=w278:T14[], "error out"=w281:errorcluster)  [unwired: 9 in]
        n125 = call "SRV_Queue_Enqueue Element at Front.vi"("error in (no error)"=w281, "Data"=w278, "Command"="Update Sensor Value", "Command-Data Queue"=w283) -> ("error out"=w280:errorcluster, "Command-Data Queue out"=w282:refnum<queue>)  [unwired: 5 in, 1 out]
      }
      frame "##&R," {
        # "Data String is everything after the Command"
        # "Pico C Shared Variable Polled"
        n126 = Unbundle By Name(w305) -> ("Polled Cfg-Cmds"=w304:T11[], "Polled Sensor View Indicator Names"=w303:T7[])
        n127 = call "SRV_Sensors Variant to Data.vi"("error in (no error)"=w307, "Data"=w309, "Command"=w308) -> ("error out"=w294:errorcluster, "Data String"=w306:string)  [unwired: 7 in]
        n128 = call "SRV_Sensor PARSE_##R.vi"("Return Data"=w306, "error in (no error)"=w294) -> ("Sensor View Indicator Names"=w302:T7, "Value"=w301:dbl, "error out"=w293:errorcluster)  [unwired: 11 in]
        n129 = call "SRV_Build Sensor-Value Cluster.vi"("Cfg-Cmds"=w304, "Sensor View Indicator Names"=w303, "Sensor View Indicator Name"=w302, "Value (for Pico C)"=w301, "error in (no error)"=w293) -> ("Array of Sensor-Value Cluster"=w295:T14[], "error out"=w298:errorcluster)  [unwired: 9 in]
        n130 = call "SRV_Queue_Enqueue Element at Front.vi"("error in (no error)"=w298, "Data"=w295, "Command"="Update Sensor Value", "Command-Data Queue"=w300) -> ("error out"=w297:errorcluster, "Command-Data Queue out"=w299:refnum<queue>)  [unwired: 5 in, 1 out]
      }
      frame "Update Sensor Value" {
        n131 = Variant To Data(error in=w317, type=T14[] [] ("Array of Sensor-Value Cluster"), Variant=w316) -> (data=w313:T14[], error out=w312:errorcluster)
        n132 = Unbundle By Name(w315) -> ("Sensor View refs"=w314:T2)
        n133 = for {
          tunnel: w314 -> [w328]
          tunnel: w313 -> [w327] mode=indexing
          shift-right: [w322] -> w311
          shift-left: w312 -> [w325]
          n134 = Unbundle By Name(w327) -> ("Sensor Name"=w326:T7, "Value"=w320:dbl)
          n135 = call "SRV_Get Sensor View ref From Selection.vi"("Sensor View refs"=w328, "Sensor View"=w326, "error in (no error)"=w325) -> ("Boolean ref?"=w321:bool, "Selected ref"=w324:refnum<vi>, "error out"=w323:errorcluster)  [unwired: 8 in, 2 out]
          n136 = case "Is Boolean ref?" shown="True" w321 {
            tunnel: w320 -> [w330 w333]
            tunnel: [w329 w331] -> w319
            frame False {
              n137 = To Variant(anything=w330) -> (Variant=w329:variant)
            }
            frame True {
              n138 = call "SRV_Is Greater Than Zero.vi"("Numeric (DBL)"=w333) -> ("Greater Than Zero"=w332:bool)  [unwired: 14 in]
              n139 = To Variant(anything=w332) -> (Variant=w331:variant)
            }
          }
          n140 = property class="Ctl"(reference=w324, error in=w323, "Value"=w319) -> (error out=w322:errorcluster)  [unwired: 1 out]
        }
      }
      frame "Developer Error", Default {
        # "generates an error with a useful message when an undefined state is requested"
        n141 = Format Into String(format string="Developer Error: the case \"%s\" is undefined.", w338) -> (resulting string=w334:string)  [unwired: 2 in, 1 out]
        n142 = call "SRV_Generate Error.vi"("Message"=w334, "error in (no error)"=w336) -> ("error out"=w335:errorcluster)  [unwired: 13 in]
      }
      frame "Error" {
        w341 = T15 1 items=["no dialog", "OK message", "continue or stop message", "OK message + warnings", "continue/stop + warnings"] ("type of dialog (OK msg:1)")
        # "Use Default If Unwired because in the other cases empty string is the same as wiring \"Error\" in the Error-State Controller VI"
        # "append the recent command history to the error souce string"
        n143 = call "SRV_Format Command History String.vi"("Command History"=w348) -> ("Command History String"=w344:string)  [unwired: 14 in]
        n144 = call "SRV_Append to New Error Source String.vi"("Message String to append"=w344, "Error In (no error)"=w345) -> ("error out"=w343:errorcluster)  [unwired: 13 in]
        n145 = call <vilib>:"General Error Handler.vi"("type of dialog (OK msg:1)"=w341, "error in (no error)"=w343) -> ("error out"=w342:errorcluster)  [unwired: 9 in, 4 out]
      }
      frame "Exit", "Exit_QueueError" {
        n146 = call "SRV_VIG_Sensor View Tab Open.vi"("Sensor View Tab Open"=FALSE, "Method (Get)"=enum16{"Get", "Set"}."Set") -> ("error out"=w353:errorcluster)  [unwired: 12 in, 1 out]
        n147 = Unbundle By Name(w358) -> ("SRV ref"=w355:refnum<k5>, "Streaming Cfg-Cmds"=w357:T11[])
        n148 = call "SRV_Sensor Streaming Sensors Off.vi"("Previous Streaming Cfg-Cmds"=w357, "error in (no error)"=w353) -> ("Streaming Cfg-Cmds OFF"=w354:T11[], "error out"=w356:errorcluster)  [unwired: 12 in]
        n149 = call "SRV_Write Sensor Commands.vi"("SRV In"=w355, "Sensor Cfg-Commands"=w354, "error in (no error)"=w356) -> ("error out"=w350:errorcluster)  [unwired: 11 in, 1 out]
        n150 = Select(t=w352, s=w352, f=w350) -> (s? t:f=w351:errorcluster)
      }
    }
    n151 = call "SRV_Command Queue Error-State Controller.vi"("error in (no error)"=w104, "Error Command"=w98, "Command-Data Queue"=w102) -> ("error out"=w103:errorcluster, "Command-Data Queue out"=w101:refnum<queue>)  [unwired: 7 in]
  }
  n152 = while {
    shift-right: [w367] -> w85
    shift-left: w87 -> [w368]
    tunnel: w4 -> [w366]
    tunnel: w88 -> [w365]
    tunnel: [w364] -> w86
    stop <- w363 stop-if-true
    n153 = event shown="[0] \"Poll\": Value Change" {
      selector: w365 -> [_ _]
      dyn-events: [_ _] -> w364
      timeout: _ -> [_ _]
      tunnel: w368 -> [w370 w374]
      tunnel: [w371 w374] -> w367
      tunnel: w366 -> [w369 _]
      tunnel: [_ TRUE] -> w363
      event "Poll": Value Change {
        n154 = event-data() -> ()  [unwired: 1 in, 5 out]
        n155 = call "SRV_Queue_Enqueue Element.vi"("error in (no error)"=w370, "Command"="Poll", "Command-Data Queue"=w369) -> ("error out"=w371:errorcluster)  [unwired: 6 in, 2 out]
      }
      event User Event {
        n156 = event-data() -> ()  [unwired: 1 in, 1 out]
      }
    }
  }
  n157 = Unregister For Events(event registration refnum=w86, error in=w85) -> (error out=w75:errorcluster)
  n158 = Unbundle By Name(w80) -> ("Make All Visible"=w1:bool, "This VI ref"=w15:refnum<vi>, "user event"=w79:refnum<user-event>)
  n159 = Release Queue(queue=w83, force destroy? (F)=TRUE, error in (no error)=w84) -> (error out=w78:errorcluster)  [unwired: 2 out]
  n160 = call "SRV_Generate User Exit Event.vi"("error in (no error)"=w78, "User Exit Event"=w79) -> ("error out"=w76:errorcluster, "User Exit Event out"=w77:refnum<user-event>)  [unwired: 8 in]
  n161 = Build Array(w76, w75) -> (w71:errorcluster[])
  n162 = Merge Errors(w71) -> (w74:errorcluster)
  n163 = Destroy User Event(user event=w77, error in=w74) -> (error out=w17:errorcluster)
  n164 = flat-sequence {
    tunnel: w17 -> [w379]
    tunnel: [w379] -> w16
    tunnel: w15 -> [w378]
    tunnel: w1 -> [w375]
    frame #0 {
      n165 = Compound Arithmetic op=AND(TRUE, invert w375) -> (w377:bool)
      n166 = case shown="True" w377 {
        tunnel: w378 -> [_ w381]
        frame False {
        }
        frame True {
          n167 = invoke class="VI" method="FP.Close"(reference=w381) -> (error out=w380:errorcluster)  [unwired: 2 in, 2 out]
          n168 = call <vilib>:"Clear Errors.vi"("error in (no error)"=w380) -> ()  [unwired: 5 in, 2 out]
        }
      }
    }
  }
  "error out" <- w16
